vi "VisualizeC37.118 PMU.vi"() -> ()   [LabVIEW 2018, in "Visualization.lvlib" / "VisualizeSensor.lvclass"]
doc: "This VI listens for any measurement data associated with the provided PluginName and displays it to the user for analysis. The display is only suitable for data coming from the RoomAlert Plugin."
uses:
  VisualizeSensor.lvclass
  Sensor/SensorShared/clSensorData.ctl
  <vilib>/event_ctls.llb/usereventprio.ctl
  VisualizeBase/VisualizeBase_class/Requests/clUserEventType.ctl
  SubVI/VisulaizationManagement/PopInOutButton.ctl
  <extravilib>/ChannelInstances/Tag-bool/Write With Abort.vi
  <extravilib>/ChannelInstances/Tag-bool/Read With Abort.vi
  <extravilib>/ChannelInstances/Tag-bool/Instantiate.vi
  <extravilib>/ChannelInstances/Tag-bool/EndpointRead.vi
  <vilib>/Utility/error.llb/Error Cluster From Error Code.vi
  <extravilib>/ChannelInstances/Tag-bool/Endpoint.vi
  <vilib>/ErrorRing/Error Ring.xnode
  <userlib>/NIST/NISTErrorLib/NISTErrorLib.lvlib
  VisualizeBase/VisualizeBase_class/VisualizeBase.lvclass
  Sensor/SensorShared/SensorShared.lvlib
  Sensor/SensorModule/SensorModule.lvlib
  <extravilib>/ChannelInstances/Tag-bool.lvlib
  TestClass/Test.lvclass
  Queue/Queue.lvlib
panel:
  in  "ModuleID":i32
  in  "Log Data":bool
  in  "btnStop":bool
  in  "btnReset":bool
  in  "btnClearTest":bool
  out "Siemens":waveform(dbl)[](graph)=[{"t0"=timestamp(3657200531.6397257 s since 1904-01-01), "dt"=1.0, "Y"=[46.19]}, {"t0"=timestamp(3657200531.6397257 s since 1904-01-01), "dt"=1.0, "Y"=[2.0]}, {"t0"=timestamp(3657200531.6397257 s since 1904-01-01), "dt"=1.0, "Y"=[60.0]}]
  out "LightTower":T1
  out "ErrorArray":errorcluster[](array[cluster])
  out "Incorrect DataType?":bool
  out "String Results":string="Sensor.RoomAlert1"
  in  "PluginName":string="Sensor.RoomAlert1"
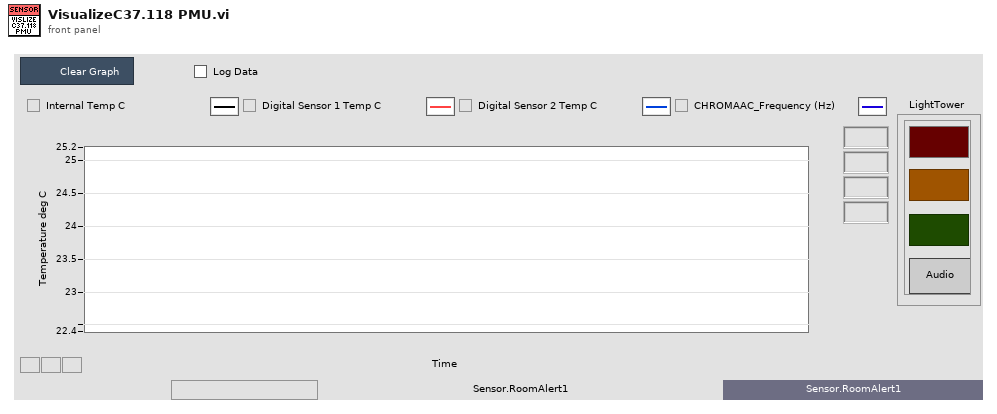
[diagram p1: front panel]
types:
  T1 = cluster{"Red":bool, "Amber":bool, "Green":bool, "Audio":bool}
  T2 = enum16{"open", "open or create", "create or replace", "create", "open (read-only)"}
  T3 = typedef "Visualization.lvlib/VisualizeBase.lvclass/clRequestEvents.ctl" = cluster{"StopRequest":refnum<user-event>, "ResetRequest":refnum<user-event>}
  T4 = typedef "SensorShared.lvlib/clBroadcastEvents.ctl" = cluster{"DidInit":refnum<user-event>, "StatusUpdate":refnum<user-event>, "ErrorReport":refnum<user-event>, "DidStop":refnum<user-event>, "PathToINI":refnum<user-event>, "SensorReport":refnum<user-event>, "SensorConfig":refnum<user-event>}
  T5 = typedef "SensorShared.lvlib/clSensorData.ctl" = cluster{"SensorType":string, "SensorData":variant}
  T6 = typedef "Visualization.lvlib/VisualizeBase.lvclass/clUserEventType.ctl" = cluster{"BusIndex":i8, "Data":variant}
  T7 = typedef "usereventprio.ctl" = enum32{"high priority", "normal priority"}
  T8 = cluster{"Red":bool, "Amber":bool, "Green":bool, "Audio":bool}[]
  T9 = typedef "Tag-bool.lvlib/))Channel.ctl" = refnum<queue>
  T10 = typedef "PopInOutButton.ctl" = bool
  T11 = cluster{"Module Name":string, "In SubPanel?":T10}
  T12 = typedef "sizeaction.ctl" = enum32{"Minimized", "Maximized", "Resized"}
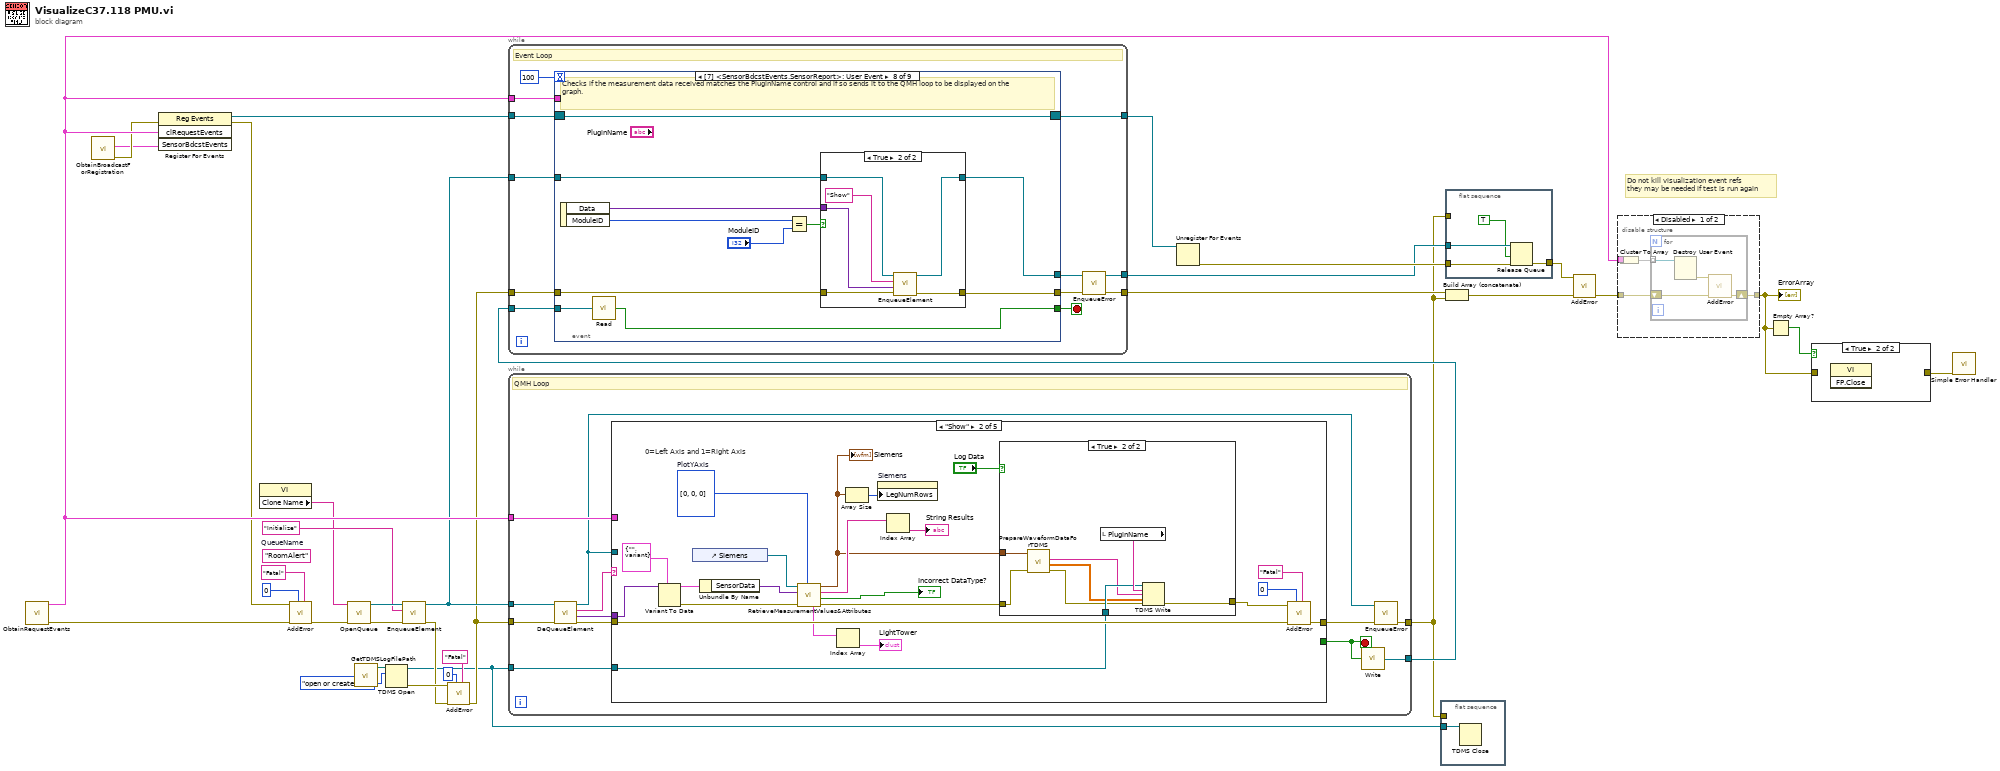
[diagram p0: block diagram]
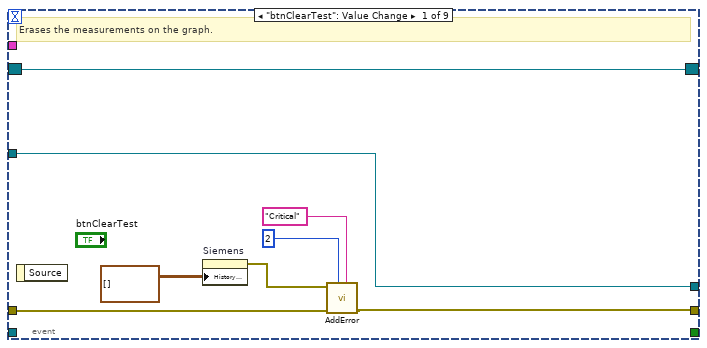
[diagram p3: hidden frame]
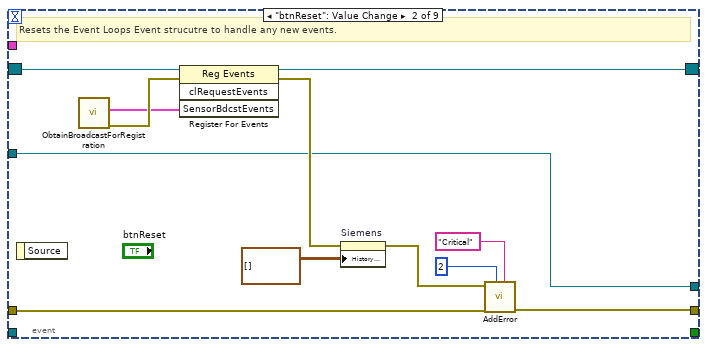
[diagram p4: hidden frame]
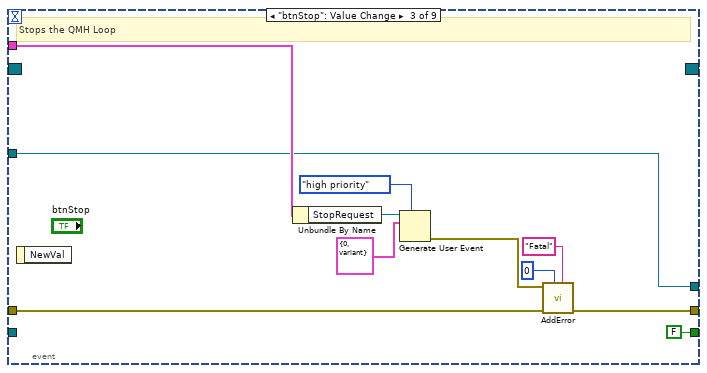
[diagram p5: hidden frame]
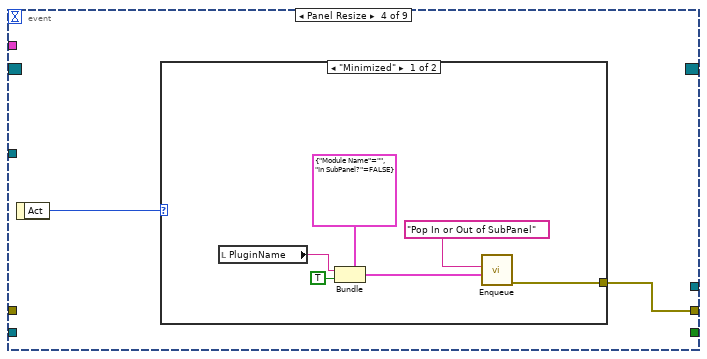
[diagram p6: hidden frame]
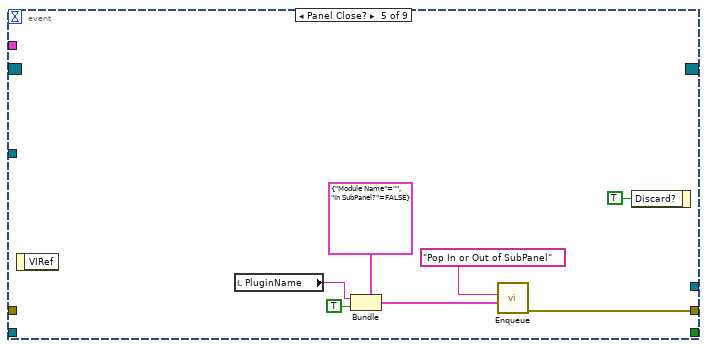
[diagram p8: hidden frame]
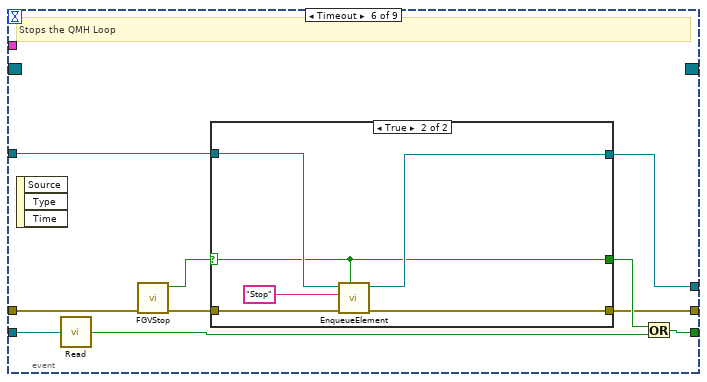
[diagram p9: hidden frame]
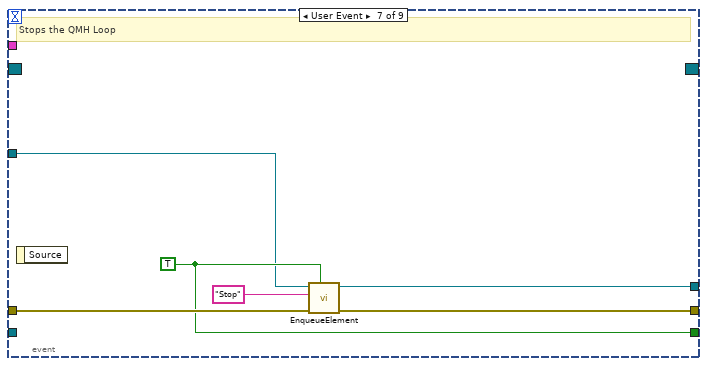
[diagram p11: hidden frame]
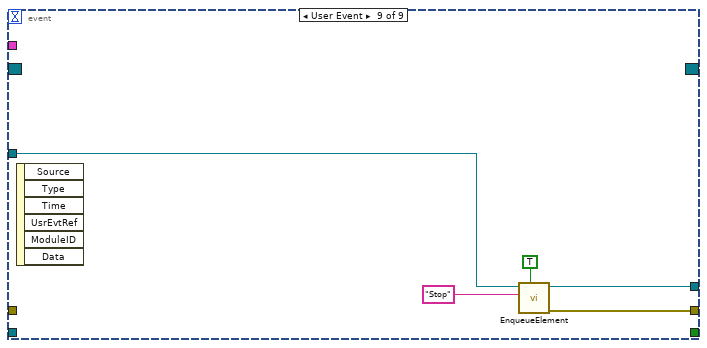
[diagram p13: hidden frame]
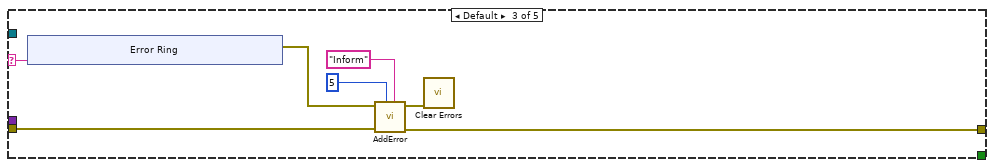
[diagram p16: hidden frame]
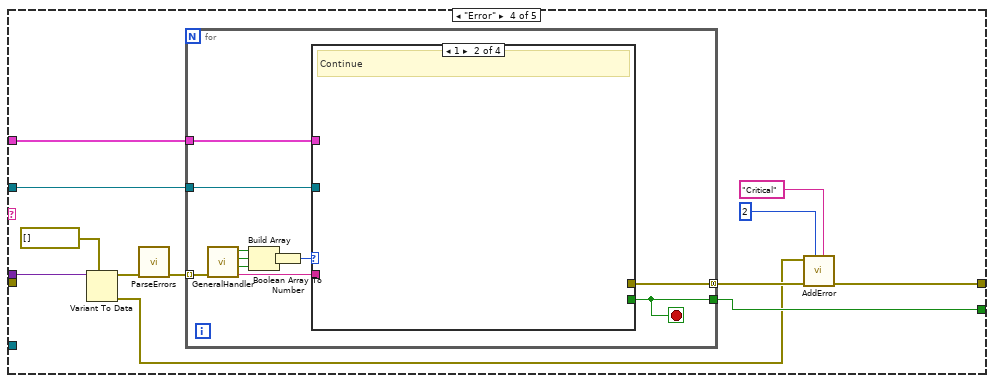
[diagram p17: hidden frame]
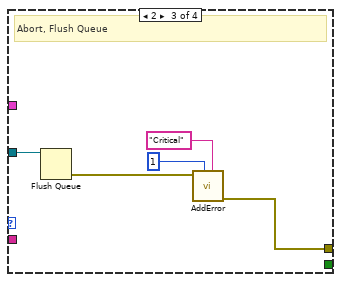
[diagram p19: hidden frame]
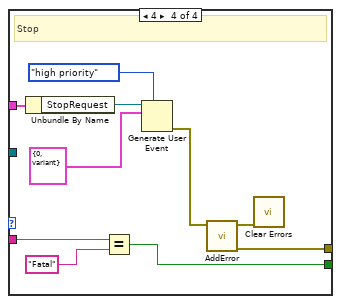
[diagram p20: hidden frame]
diagram:
  (unwired) "RoomAlert"  # QueueName
  # "Do not kill visualization event refs\nthey may be needed if test is run again"
  n1 = call "ObtainRequestEvents.vi"() -> ("Error"=w25:errorcluster[], "clRequestEvents"=w27:T3)  [unwired: 10 in]
  n2 = call "ObtainBroadcastForRegistration.vi"() -> ("error out"=w21:errorcluster, "SensorBdcstEvents"=w12:T4)  [unwired: 10 in]
  n3 = register-events(error in=w21, w27, w12) -> (reference out=w34:refnum<event-registration>, error out=w24:errorcluster)  [unwired: 1 in]
  n4 = property class="VI"() -> ("Clone Name"=w10:string)  [unwired: 2 in, 2 out]
  n5 = call <userlib>:"AddError.vi"("Severity"="Fatal", "Priority"=u8 0, "ErrorArray In"=w25, "error in (no error)"=w24) -> ("ErrorArray Out"=w20:errorcluster[])  [unwired: 6 in, 1 out]
  n6 = call "OpenQueue.vi"("Error Array In"=w20, "QueueName"=w10) -> ("Error Array Out"=w18:errorcluster[], "queue out"=w19:refnum<queue>)  [unwired: 8 in]
  n7 = call "GetTDMSLogFilePath.vi"() -> ("TDMS Log File Path"=w9:path)  [unwired: 11 in]
  n8 = TDMS Open(10:T2."open or create" ("operation (0:open)"), 11:w9) -> (0:w6:errorcluster, 3:w2:refnum<k34>)  [unwired: 5 in]
  n9 = call "EnqueueElement.vi"("Error Array In"=w18, "Message"="Initialize", "queue in"=w19) -> ("Error Array Out"=w5:errorcluster[], "queue out"=w16:refnum<queue>)  [unwired: 7 in]
  n10 = call <userlib>:"AddError.vi"("Severity"="Fatal", "Priority"=u8 0, "ErrorArray In"=w5, "error in (no error)"=w6) -> ("ErrorArray Out"=w4:errorcluster[])  [unwired: 6 in, 1 out]
  n11 = while {
    tunnel: w4 -> [w40]
    tunnel: [w43] -> w1
    tunnel: w16 -> [w39]
    tunnel: w27 -> [w45]
    tunnel: [w36] -> w11
    tunnel: w2 -> [w35]
    stop <- w46 stop-if-true
    # "QMH Loop"
    n12 = call "DeQueueElement.vi"("Error Array In"=w40, "Queue In"=w39) -> ("Error Array Out"=w38:errorcluster[], "Data"=w41:variant, "Message"=w42:string, "Queue Out"=w37:refnum<queue>)  [unwired: 6 in]
    n13 = case shown="\"Show\"" w42 {
      selector: w42 -> [_ _ w85 _ _]
      tunnel: w41 -> [_ w64 _ w104 _]
      tunnel: w38 -> [w47 w67 w83 _ w131]
      tunnel: [w47 w69 w82 w94 w131] -> w44
      tunnel: [_ _ _ w100 TRUE] -> w46
      tunnel: w45 -> [_ _ _ w99 _]
      tunnel: w37 -> [_ _ _ w98 _]
      tunnel: w35 -> [_ w55 _ _ _]
      frame "Initialize" {
      }
      frame "Show" {
        w61 = u32[] [0, 0, 0]  # PlotYAxis
        # "0=Left Axis and 1=Right Axis"
        n14 = Variant To Data(type=T5 {"SensorType"="", "SensorData"=variant} ("clSensorData"), Variant=w64) -> (data=w62:T5, error out=w63:errorcluster)  [unwired: 1 in]
        n15 = control-ref of="Siemens"() -> (w68:refnum<vi>)
        n16 = Unbundle By Name(w62) -> ("SensorData"=w59:variant)
        n17 = call "RetrieveMeasurementValues&Attributes.vi"("PlotYScale"=w61, "error in (no error)"=w63, "Variant"=w59, "WaveformChartReference"=w68) -> ("error out"=w58:errorcluster, "Incorrect DataType?"=→"Incorrect DataType?":bool, "Array Of Strings"=w54:string[], "WaveformArrayOut"=w48:waveform(dbl)[], "LightTower"=w52:T8)  [unwired: 3 in]
        "Siemens" <- w48
        n18 = Index Array(array=w52) -> (element=→"LightTower":T1)  [unwired: 1 in]
        n19 = Array Size(array=w48) -> (size(s)=w49:i32)
        n20 = property on="Siemens" class="WFChart (strict)"("LegNumRows"=w49) -> ()  [unwired: 2 in, 2 out]
        n21 = Index Array(array=w54) -> (element=→"String Results":string)  [unwired: 1 in]
        n22 = case shown="True" "Log Data" {
          tunnel: w58 -> [w70 w77]
          tunnel: [w70 w78] -> w57
          tunnel: w48 -> [_ w76]
          tunnel: w55 -> [_ w74]
          frame False {
          }
          frame True {
            n23 = call "PrepareWaveformDataForTDMS.vi"("error in (no error)"=w77, "WaveformArray in"=w76) -> ("error out"=w73:errorcluster, "Measurement Data"=w71:dbl[][], "Channel Names"=w72:string[])  [unwired: 7 in]
            n24 = local read "PluginName"() -> (w75:string)
            n25 = TDMS Write(0:w74, 5:w75, 7:w72, 9:w71, 11:w73) -> (15:w78:errorcluster)  [unwired: 1 in, 3 out]
          }
        }
        n26 = call <userlib>:"AddError.vi"("Severity"="Fatal" ("String"), "Priority"=u8 0, "ErrorArray In"=w67, "error in (no error)"=w57) -> ("ErrorArray Out"=w69:errorcluster[])  [unwired: 6 in, 1 out]
      }
      frame Default {
        n27 = xnode "Error Ring"("parameter 0"=w85) -> ("error out"=w84:errorcluster)
        n28 = call <userlib>:"AddError.vi"("Severity"="Inform" ("String"), "Priority"=u8 5, "ErrorArray In"=w83, "error in (no error)"=w84) -> ("ErrorArray Out"=w82:errorcluster[], "error out"=w81:errorcluster)  [unwired: 6 in]
        n29 = call <vilib>:"Clear Errors.vi"("error in (no error)"=w81) -> ()  [unwired: 5 in, 2 out]
      }
      frame "Error" {
        n30 = Variant To Data(type=errorcluster[] [], Variant=w104) -> (data=w102:errorcluster[], error out=w93:errorcluster)  [unwired: 1 in]
        n31 = call <userlib>:"ParseErrors.vi"("ErrorArray"=w102) -> ("ErrorArray"=w101:errorcluster[])  [unwired: 8 in, 2 out]
        n32 = for {
          tunnel: w101 -> [w115] mode=indexing
          tunnel: [w109] -> w95 mode=concatenating
          tunnel: [w107] -> w100
          tunnel: w99 -> [w106]
          tunnel: w98 -> [w105]
          stop <- w107 stop-if-true
          n33 = call <userlib>:"GeneralHandler.vi"("error in (no error)"=w115) -> ("Severity"=w108:string, "Stop"=w112:bool, "Abort"=w113:bool, "Continue"=w114:bool)  [unwired: 6 in, 1 out]
          n34 = Build Array(w114, w113, w112) -> (w111:bool[])
          n35 = Boolean Array To Number(Boolean array=w111) -> (number=w110:u32)
          n36 = case shown="1" w110 {
            tunnel: [_ _ w120 w129] -> w109
            tunnel: w108 -> [_ _ _ w122]
            tunnel: [_ _ _ w124] -> w107
            tunnel: w106 -> [_ _ _ w123]
            tunnel: w105 -> [_ _ w116 _]
            frame 0, Default {
              # "No Dialog"
            }
            frame 1 {
              # "Continue"
            }
            frame 2 {
              # "Abort, Flush Queue"
              n37 = Flush Queue(queue=w116) -> (error out=w119:errorcluster)  [unwired: 1 in, 2 out]
              n38 = call <userlib>:"AddError.vi"("Severity"="Critical" ("String"), "Priority"=u8 1, "error in (no error)"=w119) -> ("ErrorArray Out"=w120:errorcluster[])  [unwired: 7 in, 1 out]
            }
            frame 4 {
              # "Stop"
              n39 = Unbundle By Name(w123) -> ("StopRequest"=w130:refnum<user-event>)
              n40 = Equal?(x=w122, y="Fatal" ("x")) -> (x = y?=w124:bool)
              n41 = Generate User Event(priority (normal)=usereventprio."high priority", user event=w130, event data cluster=T6 {"BusIndex"=0, "Data"=variant} ("event data")) -> (error out=w128:errorcluster)  [unwired: 1 in, 1 out]
              n42 = call <userlib>:"AddError.vi"("error in (no error)"=w128) -> ("ErrorArray Out"=w129:errorcluster[], "error out"=w125:errorcluster)  [unwired: 9 in]
              n43 = call <vilib>:"Clear Errors.vi"("error in (no error)"=w125) -> ()  [unwired: 5 in, 2 out]
            }
          }
        }
        n44 = call <userlib>:"AddError.vi"("Severity"="Critical", "Priority"=u8 2, "ErrorArray In"=w95, "error in (no error)"=w93) -> ("ErrorArray Out"=w94:errorcluster[])  [unwired: 6 in, 1 out]
      }
      frame "Stop" {
      }
    }
    n45 = call <extravilib>:"Write.vi"("element"=w46) -> ("channel"=w36:T9)  [unwired: 1 out]
    n46 = call "EnqueueError.vi"("Error Array In"=w44, "Queue in"=w37) -> ("Error Array Out"=w43:errorcluster[])  [unwired: 8 in, 1 out]
  }
  n47 = while {
    tunnel: w34 -> [w144]
    tunnel: [w138] -> w32
    tunnel: [w142] -> w33
    tunnel: w27 -> [w141]
    tunnel: w4 -> [w140]
    tunnel: w16 -> [w139]
    tunnel: [w135] -> w15
    tunnel: w11 -> [w133]
    stop <- w143 stop-if-true
    # "Event Loop"
    n48 = event shown="[7] <SensorBdcstEvents.SensorReport>: User Event" {
      selector: w144 -> [w146 w164 _ _ _ _ _ w222 _]
      dyn-events: [w146 w163 _ _ _ _ _ w222 _] -> w142
      timeout: 100 -> [_ _ _ _ _ _ _ _ _]
      tunnel: [_ _ FALSE ("Priority? (F)") _ _ w191 w212 w219 _] -> w143
      tunnel: [w149 w161 w168 w176 w190 w193 w214 w224 w237] -> w137
      tunnel: w141 -> [_ _ w167 _ _ _ _ _ _]
      tunnel: w140 -> [w150 w162 w175 _ _ w196 w215 w225 _]
      tunnel: w139 -> [w145 w154 w165 _ _ w195 w210 w226 w235]
      tunnel: [w145 w154 w165 _ _ w194 w213 w223 w236] -> w136
      tunnel: w133 -> [_ _ _ _ _ w200 _ w220 _]
      event "btnClearTest": Value Change {
        # "Erases the measurements on the graph."
        n49 = event-data() -> ()  [unwired: 1 in, 1 out]
        n50 = property on="Siemens" class="WFChart (strict)"("History Data"=waveform(dbl)[][] []) -> (error out=w148:errorcluster)  [unwired: 2 in, 1 out]
        n51 = call <userlib>:"AddError.vi"("Severity"="Critical", "Priority"=u8 2, "ErrorArray In"=w150, "error in (no error)"=w148) -> ("ErrorArray Out"=w149:errorcluster[])  [unwired: 6 in, 1 out]
      }
      event "btnReset": Value Change {
        # "Resets the Event Loops Event strucutre to handle any new events."
        n52 = event-data() -> ()  [unwired: 1 in, 1 out]
        n53 = call "ObtainBroadcastForRegistration.vi"() -> ("error out"=w155:errorcluster, "SensorBdcstEvents"=w153:T4)  [unwired: 10 in]
        n54 = register-events(reference=w164, error in=w155, w153) -> (reference out=w163:refnum<event-registration>, error out=w157:errorcluster)  [unwired: 1 in]
        n55 = property on="Siemens" class="WFChart (strict)"(error in=w157, "History Data"=waveform(dbl)[][] []) -> (error out=w156:errorcluster)  [unwired: 1 in, 1 out]
        n56 = call <userlib>:"AddError.vi"("Severity"="Critical", "Priority"=u8 2, "ErrorArray In"=w162, "error in (no error)"=w156) -> ("ErrorArray Out"=w161:errorcluster[])  [unwired: 6 in, 1 out]
      }
      event "btnStop": Value Change {
        # "Stops the QMH Loop"
        n57 = event-data() -> ()  [unwired: 1 in, 1 out]
        n58 = Unbundle By Name(w167) -> ("StopRequest"=w173:refnum<user-event>)
        n59 = Generate User Event(priority (normal)=usereventprio."high priority", user event=w173, event data cluster=T6 {"BusIndex"=0, "Data"=variant} ("event data")) -> (error out=w174:errorcluster)  [unwired: 1 in, 1 out]
        n60 = call <userlib>:"AddError.vi"("Severity"="Fatal" ("String"), "Priority"=u8 0, "ErrorArray In"=w175, "error in (no error)"=w174) -> ("ErrorArray Out"=w168:errorcluster[])  [unwired: 6 in, 1 out]
      }
      event Panel Resize {
        n61 = event-data() -> ("Act"=w177:T12)  [unwired: 1 in]
        n62 = case shown="\"Minimized\"" w177 {
          tunnel: [w178 _] -> w176
          frame "Minimized" {
            n63 = local read "PluginName"() -> (w180:string)
            n64 = Bundle(cluster=T11 {"Module Name"="", "In SubPanel?"=FALSE} ("output cluster"), "Module Name"=w180, "In SubPanel?"=T10 TRUE) -> (w182:T11)
            n65 = call "Enqueue.vi"("Message Data"=w182, "Message"="Pop In or Out of SubPanel") -> ("ErrorArray"=w178:errorcluster[])  [unwired: 9 in]
          }
          frame "Maximized", Default {
          }
        }
      }
      event Panel Close? {
        n66 = event-data() -> ()  [unwired: 1 in, 1 out]
        n67 = local read "PluginName"() -> (w186:string)
        n68 = Bundle(cluster=T11 {"Module Name"="", "In SubPanel?"=FALSE} ("output cluster"), "Module Name"=w186, "In SubPanel?"=T10 TRUE) -> (w188:T11)
        n69 = call "Enqueue.vi"("Message Data"=w188, "Message"="Pop In or Out of SubPanel") -> ("ErrorArray"=w190:errorcluster[])  [unwired: 9 in]
        n70 = event-data("Discard?"=TRUE) -> ()  [unwired: 1 in, 1 out]
      }
      event Timeout {
        # "Stops the QMH Loop"
        n71 = event-data() -> ()  [unwired: 1 in, 3 out]
        n72 = call <extravilib>:"Read.vi"("channel"=w200) -> ("element"=w192:bool)  [unwired: 1 in, 1 out]
        n73 = call "FGVStop.vi"("Error In"=w196) -> ("Error Out"=w198:errorcluster[], "Value"=w199:bool)  [unwired: 9 in]
        n74 = case shown="True" w199 {
          selector: w199 -> [w201 w204]
          tunnel: [w203 w207] -> w193
          tunnel: w198 -> [w203 w208]
          tunnel: w195 -> [w202 w206]
          tunnel: [w202 w205] -> w194
          tunnel: [w201 w204] -> w197
          frame False {
          }
          frame True {
            n75 = call "EnqueueElement.vi"("Priority? (F)"=w204, "Error Array In"=w208, "Message"="Stop", "queue in"=w206) -> ("Error Array Out"=w207:errorcluster[], "queue out"=w205:refnum<queue>)  [unwired: 6 in]
          }
        }
        n76 = Or(x=w197, y=w192) -> (x .or. y?=w191:bool)
      }
      event User Event {
        w212 = TRUE ("Priority? (F)")
        # "Stops the QMH Loop"
        n77 = event-data() -> ()  [unwired: 1 in, 1 out]
        n78 = call "EnqueueElement.vi"("Priority? (F)"=w212, "Error Array In"=w215, "Message"="Stop", "queue in"=w210) -> ("Error Array Out"=w214:errorcluster[], "queue out"=w213:refnum<queue>)  [unwired: 6 in]
      }
      event User Event {
        # "Checks if the measurement data received matches the PluginName control and if so sends it to the QMH loop to be displayed on the graph."
        n79 = event-data() -> ("Data"=w221:variant, "ModuleID"=w216:i32)  [unwired: 1 in]
        n80 = call <extravilib>:"Read.vi"("channel"=w220) -> ("element"=w219:bool)  [unwired: 1 in, 1 out]
        n81 = Equal?(x=w216, y="ModuleID") -> (x = y?=w218:bool)
        n82 = case shown="True" w218 {
          tunnel: [w227 w233] -> w224
          tunnel: w226 -> [w228 w232]
          tunnel: w225 -> [w227 w234]
          tunnel: [w228 w230] -> w223
          tunnel: w221 -> [_ w231]
          frame False {
          }
          frame True {
            n83 = call "EnqueueElement.vi"("Error Array In"=w234, "Data"=w231, "Message"="Show", "queue in"=w232) -> ("Error Array Out"=w233:errorcluster[], "queue out"=w230:refnum<queue>)  [unwired: 6 in]
          }
        }
      }
      event User Event {
        n84 = event-data() -> ()  [unwired: 1 in, 6 out]
        n85 = call "EnqueueElement.vi"("Priority? (F)"=TRUE, "Message"="Stop", "queue in"=w235) -> ("Error Array Out"=w237:errorcluster[], "queue out"=w236:refnum<queue>)  [unwired: 7 in]
      }
    }
    n86 = call "EnqueueError.vi"("Error Array In"=w137, "Queue in"=w136) -> ("Error Array Out"=w138:errorcluster[], "Queue out"=w135:refnum<queue>)  [unwired: 8 in]
  }
  n87 = Unregister For Events(event registration refnum=w33) -> (error out=w31:errorcluster)  [unwired: 1 in]
  n88 = flat-sequence {
    tunnel: w2 -> [w240]
    tunnel: w1 -> [_]
    frame #0 {
      n89 = TDMS Close(11:w240) -> ()  [unwired: 1 in, 2 out]
    }
  }
  n90 = flat-sequence {
    tunnel: w31 -> [w244]
    tunnel: [w243] -> w29
    tunnel: w15 -> [w242]
    tunnel: w1 -> [_]
    frame #0 {
      n91 = Release Queue(queue=w242, force destroy? (F)=TRUE, error in (no error)=w244) -> (error out=w243:errorcluster)  [unwired: 2 out]
    }
  }
  n92 = Build Array (concatenate)(w32, w1) -> (w30:errorcluster[])
  n93 = call <userlib>:"AddError.vi"("ErrorArray In"=w30, "error in (no error)"=w29) -> ("ErrorArray Out"=w28:errorcluster[])  [unwired: 8 in, 1 out]
  n94 = disable-structure shown="Disabled" {
    disable-tunnel: w28 -> [w247 w253]
    disable-tunnel: w27 -> [w246 _]
    disable-tunnel: [w245 w253] -> w14
    frame Disabled {
      n95 = Cluster To Array(cluster=w246) -> (array=w248:refnum<user-event>[])
      n96 = for {
        tunnel: w248 -> [w252] mode=indexing
        shift-right: [w251] -> w245
        shift-left: w247 -> [w250]
        n97 = Destroy User Event(user event=w252) -> (error out=w249:errorcluster)  [unwired: 1 in]
        n98 = call <userlib>:"AddError.vi"("ErrorArray In"=w250, "error in (no error)"=w249) -> ("ErrorArray Out"=w251:errorcluster[])  [unwired: 8 in, 1 out]
      }
    }
    frame Enabled {
    }
  }
  "ErrorArray" <- w14
  n99 = Empty Array?(array=w14) -> (empty?=w26:bool)
  n100 = case shown="True" w26 {
    tunnel: [w254 _] -> w13
    tunnel: w14 -> [w255 _]
    frame False {
      n101 = Merge Errors(w255) -> (w254:errorcluster)
    }
    frame True {
      n102 = invoke class="VI" method="FP.Close"() -> ()  [unwired: 3 in, 3 out]
    }
  }
  n103 = call <vilib>:"Simple Error Handler.vi"("error in (no error)"=w13) -> ()  [unwired: 4 in, 5 out]
